vi "get properties.vi"(8 "error in (no error)":errorcluster, 11 "LineCCD in":refnum<class "LineCCD.lvclass">) -> (0 "error out":errorcluster, 3 "LineCCD out":refnum<class "LineCCD.lvclass">)   [LabVIEW 2012, in "LineCCD.lvclass"]
uses:
  LineCCD.lvclass
  LineCCD.lvclass/LineCCD.ctl
  <instrlib>/ALPHALAS CCD S Series/ALPHALAS CCD S Series.lvlib
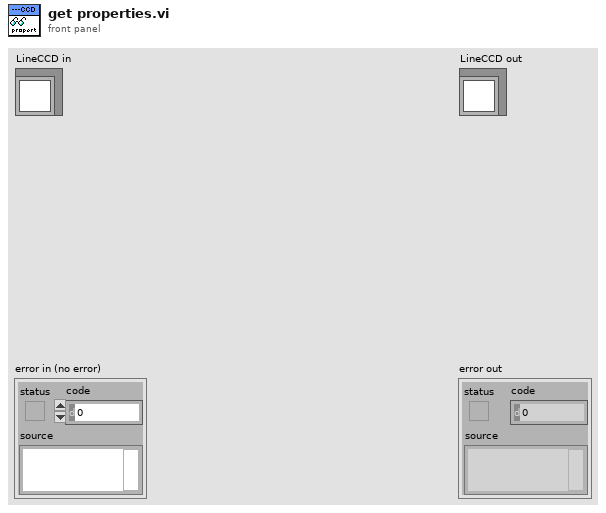
[diagram p1: front panel]
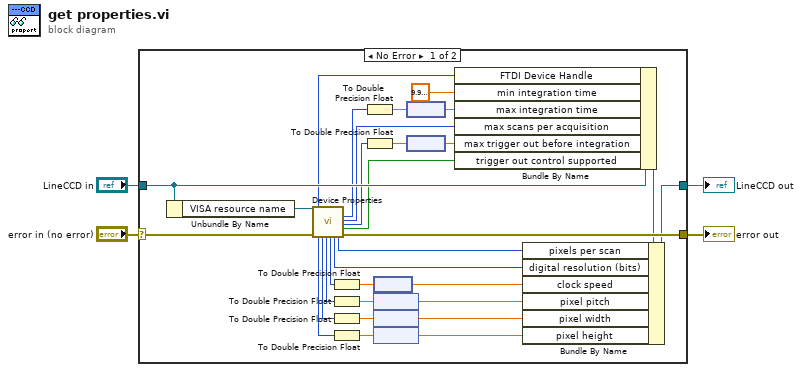
[diagram p0: block diagram]
diagram:
  n1 = case shown="No Error" "error in (no error)" {
    selector: "error in (no error)" -> [w33 w36]
    tunnel: [w32 w36] -> w3
    tunnel: [w15 w35] -> w1
    tunnel: "LineCCD in" -> [w17 w35]
    frame No Error {
      n2 = Unbundle By Name(w17) -> ("VISA resource name"=w34:refnum<visa-resource-name>)
      n3 = call <instrlib>:"Device Properties.vi"("VISA resource name"=w34, "error in (no error)"=w33) -> ("FTDI Device Handle"=w14:u32, "Sensor Pixel Height (µm)"=w31:u32, "Sensor Pixel Width (µm)"=w24:u32, "Sensor Pixel Pitch (µm)"=w23:u32, "Clock Speed (µs)"=w20:u32, "Digital Resolution (bits)"=w19:u32, "Pixels per Scan"=w18:u32, "Max Integration Time (µs)"=w12:u32, "Max Scans per Acquisition"=w11:u32, "Max Trig Out Before Integration (µs)"=w7:u32, "Trig Out Control Supported"=w6:bool, "error out"=w32:errorcluster)  [unwired: 6 in, 8 out]
      n4 = To Double Precision Float(number=w20) -> (double precision float=w22:dbl)
      n5 = To Double Precision Float(number=w23) -> (double precision float=w27:dbl)
      n6 = To Double Precision Float(number=w24) -> (double precision float=w28:dbl)
      n7 = To Double Precision Float(number=w31) -> (double precision float=w30:dbl)
      n8 = To Double Precision Float(number=w12) -> (double precision float=w13:dbl)
      n9 = To Double Precision Float(number=w7) -> (double precision float=w9:dbl)
      n10 = node(w22) -> (w21:dbl[unit])
      n11 = node(w27) -> (w25:dbl[unit])
      n12 = node(w28) -> (w26:dbl[unit])
      n13 = node(w30) -> (w29:dbl[unit])
      n14 = node(w13) -> (w10:dbl[unit])
      n15 = node(w9) -> (w8:dbl[unit])
      n16 = Bundle By Name(cluster=w17, "FTDI Device Handle"=w14, "min integration time"=dbl[unit] 9.999999999999999e-06 ("runtime.min integration time"), "max integration time"=w10, "max scans per acquisition"=w11, "max trigger out before integration"=w8, "trigger out control supported"=w6) -> (w16:refnum<class "LineCCD.lvclass">)
      n17 = Bundle By Name(cluster=w16, "pixels per scan"=w18, "digital resolution (bits)"=w19, "clock speed"=w21, "pixel pitch"=w25, "pixel width"=w26, "pixel height"=w29) -> (w15:refnum<class "LineCCD.lvclass">)
    }
    frame Error {
    }
  }
  "error out" <- w3
  "LineCCD out" <- w1
